vi "Write scrolling mode.vi"(8 "error in (no error)":errorcluster, 10 "Scrolling mode":T1, 11 "D_Datagrid in":refnum<class "D_Datagrid.lvclass">) -> (0 "error out":errorcluster, 3 "D_Datagrid out":refnum<class "D_Datagrid.lvclass">)   [LabVIEW 2023, in "D Datagrid Library.lvlib" / "D_Datagrid.lvclass"]
uses:
  D_Datagrid.lvclass
  D_Datagrid.lvclass/D_Datagrid.ctl
  Scrolling behavior.ctl
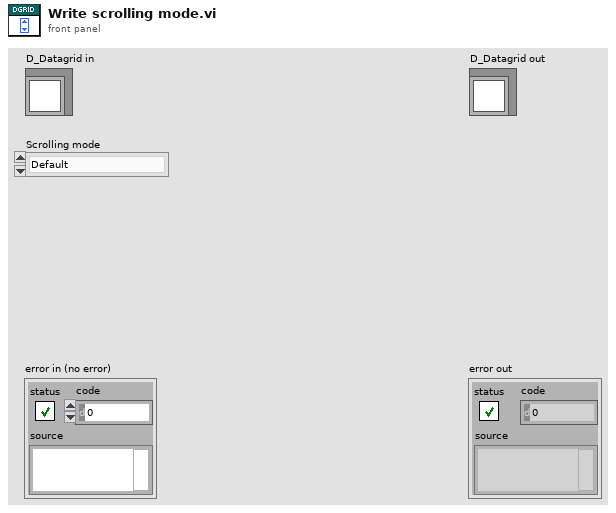
[diagram p1: front panel]
types:
  T1 = typedef "D Datagrid Library.lvlib/D_Datagrid.lvclass/Scrolling behavior.ctl" = enum16{"Default", "Locked", "Displayed items only"}
  T2 = typedef "D Datagrid Library.lvlib/D_Datagrid.lvclass/State Data.ctl" = cluster{"Data elements":refnum<class "DatagridElement.lvclass">[][], "Auto-update indicator":bool, "Scrolling mode":T1}
  T3 = enum16{"None", "On Hover", "On Key Focus", "On Hover or Key Focus"}
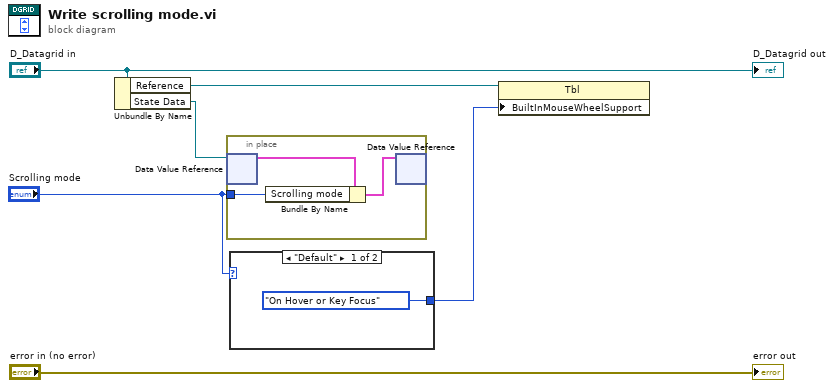
[diagram p0: block diagram]
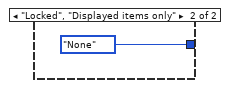
[diagram p2: hidden frame]
diagram:
  n1 = Unbundle By Name("D_Datagrid in") -> ("Reference"=w3:refnum<vi>, "State Data"=w4:refnum<data-value>)
  n2 = in-place {
    in-place-border: "Scrolling mode" -> [w7]
    n3 = in-place-dvr #1(w4) -> (w9:T2)  [unwired: 1 out]
    n4 = Bundle By Name(cluster=w9, "Scrolling mode"=w7) -> (w8:T2)
    n5 = in-place-dvr #1(w8) -> ()  [unwired: 2 out]
  }
  n6 = case shown="\"Default\"" "Scrolling mode" {
    tunnel: [T3."On Hover or Key Focus" ("Built-In Mouse Wheel Support") T3."None" ("Built-In Mouse Wheel Support")] -> w1
    frame "Default" {
    }
    frame "Locked", "Displayed items only" {
    }
  }
  n7 = property class="Tbl"(reference=w3, "BuiltInMouseWheelSupport"=w1) -> ()  [unwired: 1 in, 2 out]
  "error out" <- "error in (no error)"
  "D_Datagrid out" <- "D_Datagrid in"
